vi "RUSHShoot.vi"(1 "In Cluster":T2) -> (0 "Out Cluster":T1)   [LabVIEW 2012]
panel:
  in  "Highest POT pos":dbl=4.2
  in  "Lowest POT pos":dbl=2.1
  in  "ShootPOTToPowConst":dbl=1.0
  in  "Vision Speed Const":dbl=0.75
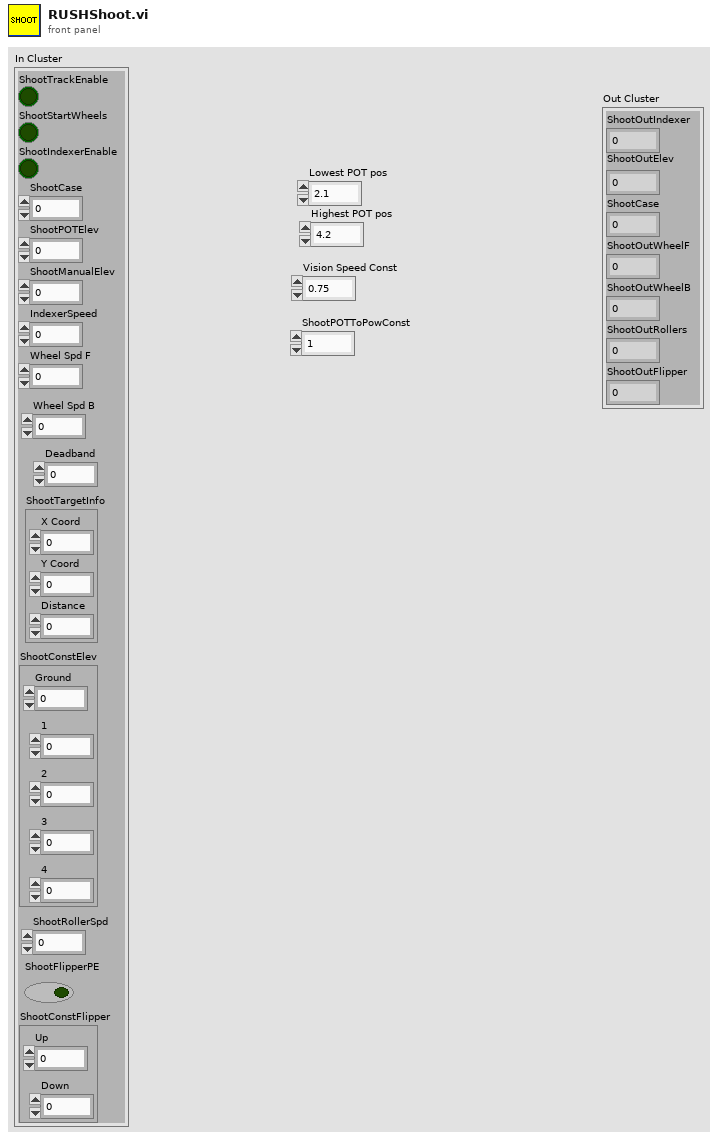
[diagram p1: front panel]
types:
  T1 = cluster{"ShootOutIndexer":dbl, "ShootOutElev":dbl, "ShootCase":dbl, "ShootOutWheelF":dbl, "ShootOutWheelB":dbl, "ShootOutRollers":dbl, "ShootOutFlipper":dbl}
  T2 = cluster{"ShootTrackEnable":bool, "ShootStartWheels":bool, "ShootIndexerEnable":bool, "ShootCase":dbl, "ShootPOTElev":dbl, "ShootManualElev":dbl, "IndexerSpeed":dbl, "Wheel Spd F":dbl, "Deadband":dbl, "ShootTargetInfo":cluster{"X Coord":dbl, "Y Coord":dbl, "Distance":dbl}, "ShootConstElev":cluster{"1":dbl, "2":dbl, "3":dbl, "4":dbl, "Ground":dbl}, "ShootRollerSpd":dbl, "ShootFlipperPE":bool, "ShootConstFlipper":cluster{"Down":dbl, "Up":dbl}, "Wheel Spd B":dbl}
  T3 = cluster{"X Coord":dbl, "Y Coord":dbl, "Distance":dbl}
  T4 = cluster{"1":dbl, "2":dbl, "3":dbl, "4":dbl, "Ground":dbl}
  T5 = cluster{"f":dbl, "y":dbl, "f":dbl, "f":dbl, "f":dbl, "f":dbl, "Down":dbl}
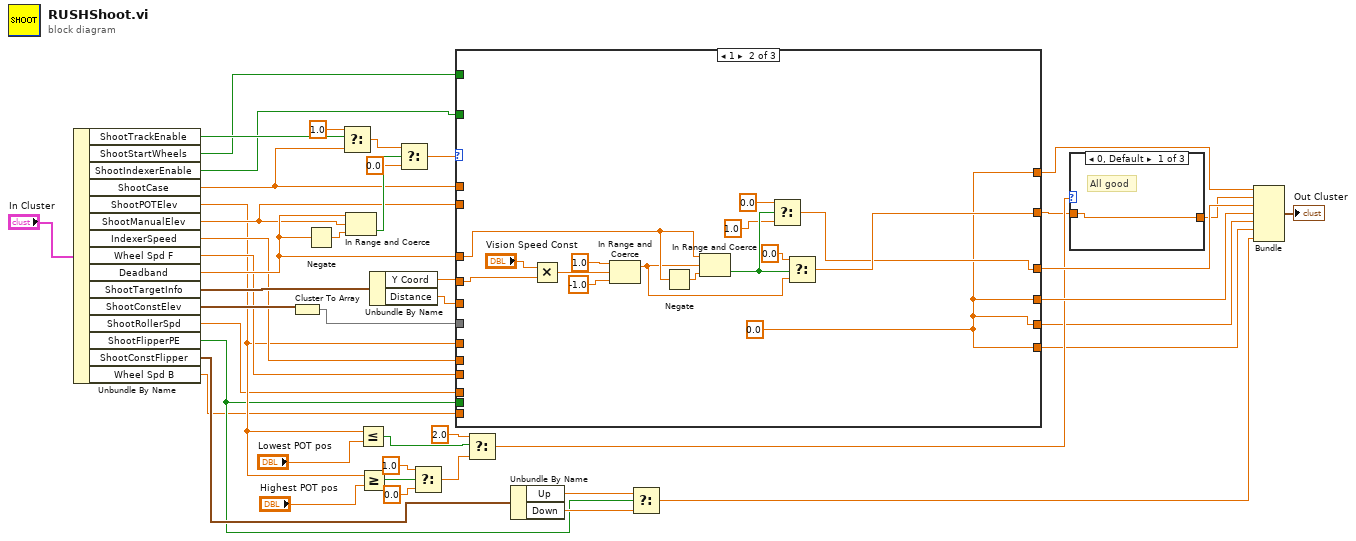
[diagram p0: block diagram]
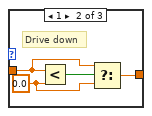
[diagram p2: hidden frame]
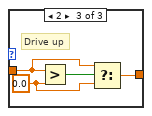
[diagram p3: hidden frame]
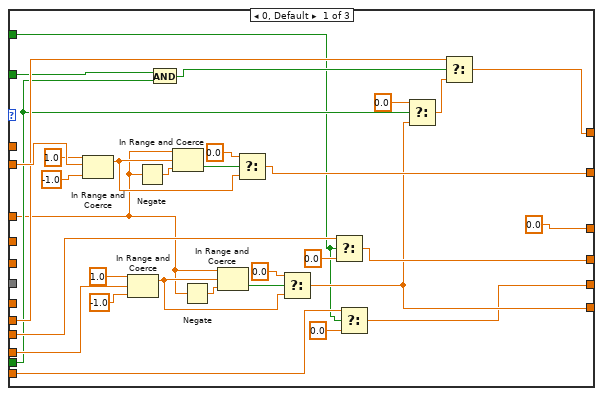
[diagram p4: hidden frame]
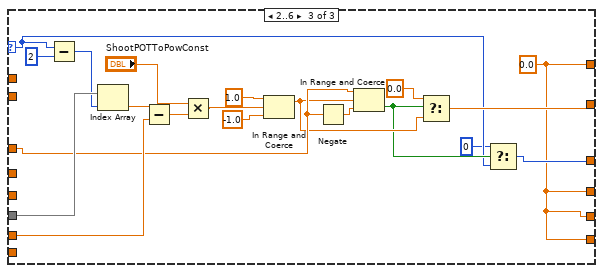
[diagram p5: hidden frame]
diagram:
  n1 = Unbundle By Name("In Cluster") -> ("ShootTrackEnable"=w44:bool, "ShootStartWheels"=w32:bool, "ShootIndexerEnable"=w31:bool, "ShootCase"=w33:dbl, "ShootPOTElev"=w21:dbl, "ShootManualElev"=w30:dbl, "IndexerSpeed"=w24:dbl, "Wheel Spd F"=w23:dbl, "Deadband"=w34:dbl, "ShootTargetInfo"=w37:T3, "ShootConstElev"=w29:T4, "ShootRollerSpd"=w10:dbl, "ShootFlipperPE"=w6:bool, "ShootConstFlipper"=w8:cluster{"Down":dbl, "Up":dbl}, "Wheel Spd B"=w5:dbl)
  n2 = Cluster To Array(cluster=w29) -> (array=w28:dbl[])
  n3 = Negate(x=w34) -> (-x=w41:dbl)
  n4 = Select(t=1.0, s=w44, f=w33) -> (s? t:f=w42:dbl)
  n5 = In Range and Coerce(upper limit=w34, x=w30, lower limit=w41) -> (In Range?=w40:bool)  [unwired: 1 out]
  n6 = Less Or Equal?(x=w21, y="Lowest POT pos") -> (x <= y?=w15:bool)
  n7 = Greater Or Equal?(x=w21, y="Highest POT pos") -> (x >= y?=w19:bool)
  n8 = Unbundle By Name(w37) -> ("Y Coord"=w36:dbl, "Distance"=w35:dbl)
  n9 = Select(t=w42, s=w40, f=0.0) -> (s? t:f=w38:dbl)
  n10 = Select(t=1.0, s=w19, f=0.0) -> (s? t:f=w16:dbl)
  n11 = case shown="1" w38 {
    selector: w38 -> [_ _ w96]
    tunnel: w36 -> [_ w91 _]
    tunnel: w35 -> [_ _ _]
    tunnel: w34 -> [w50 w86 w101]
    tunnel: [0.0 ("upper limit") w80 w94] -> w26
    tunnel: w33 -> [_ _ _]
    tunnel: [w70 w81 w98] -> w12
    tunnel: [w68 w78 w93] -> w25
    tunnel: [w77 w78 w93] -> w27
    tunnel: w32 -> [w47 _ _]
    tunnel: w31 -> [w56 _ _]
    tunnel: w30 -> [w74 _ _]
    tunnel: w28 -> [_ _ w111]
    tunnel: w21 -> [_ _ w108]
    tunnel: w24 -> [w64 _ _]
    tunnel: w23 -> [w65 _ _]
    tunnel: w10 -> [w57 _ _]
    tunnel: [w52 w78 w93] -> w3
    tunnel: w6 -> [w54 _ _]
    tunnel: w5 -> [w48 _ _]
    tunnel: [w46 w78 w93] -> w2
    frame 0, Default {
      n12 = In Range and Coerce(upper limit=1.0, x=w74, lower limit=-1.0 ("upper limit")) -> (coerced(x)=w71:dbl)  [unwired: 1 out]
      n13 = In Range and Coerce(upper limit=1.0, x=w57, lower limit=-1.0 ("upper limit")) -> (coerced(x)=w62:dbl)  [unwired: 1 out]
      n14 = Negate(x=w50) -> (-x=w75:dbl)
      n15 = And(x=w56, y=w54) -> (x .and. y?=w55:bool)
      n16 = In Range and Coerce(upper limit=w50, x=w71, lower limit=w75) -> (In Range?=w73:bool)  [unwired: 1 out]
      n17 = Negate(x=w50) -> (-x=w59:dbl)
      n18 = In Range and Coerce(upper limit=w50, x=w62, lower limit=w59) -> (In Range?=w60:bool)  [unwired: 1 out]
      n19 = Select(t=0.0, s=w73, f=w71) -> (s? t:f=w70:dbl)
      n20 = Select(t=0.0, s=w60, f=w62) -> (s? t:f=w52:dbl)
      n21 = Select(t=w65, s=w47, f=0.0 ("t")) -> (s? t:f=w68:dbl)
      n22 = Select(t=w48, s=w47, f=0.0 ("t")) -> (s? t:f=w46:dbl)
      n23 = Select(t=0.0, s=w54, f=w52) -> (s? t:f=w51:dbl)
      n24 = Select(t=w64, s=w55, f=w51) -> (s? t:f=w77:dbl)
    }
    frame 1 {
      w78 = 0.0
      n25 = Multiply(x="Vision Speed Const", y=w91) -> (x*y=w90:dbl)
      n26 = In Range and Coerce(upper limit=1.0, x=w90, lower limit=-1.0 ("upper limit")) -> (coerced(x)=w84:dbl)  [unwired: 1 out]
      n27 = Negate(x=w86) -> (-x=w87:dbl)
      n28 = In Range and Coerce(upper limit=w86, x=w84, lower limit=w87) -> (In Range?=w83:bool)  [unwired: 1 out]
      n29 = Select(t=0.0, s=w83, f=1.0) -> (s? t:f=w80:dbl)
      n30 = Select(t=0.0, s=w83, f=w84) -> (s? t:f=w81:dbl)
    }
    frame 2..6 {
      w93 = 0.0 ("f")
      n31 = Subtract(x=w96, y=2) -> (x-y=w110:i32)
      n32 = Index Array(array=w111, index=w110) -> (element=w109:dbl)
      n33 = Subtract(x=w109, y=w108) -> (x-y=w107:dbl)
      n34 = Multiply(x="ShootPOTToPowConst", y=w107) -> (x*y=w102:dbl)
      n35 = In Range and Coerce(upper limit=1.0, x=w102, lower limit=-1.0 ("upper limit")) -> (coerced(x)=w99:dbl)  [unwired: 1 out]
      n36 = Negate(x=w101) -> (-x=w103:dbl)
      n37 = In Range and Coerce(upper limit=w101, x=w99, lower limit=w103) -> (In Range?=w97:bool)  [unwired: 1 out]
      n38 = Select(t=0.0, s=w97, f=w99) -> (s? t:f=w98:dbl)
      n39 = Select(t=0, s=w97, f=w96) -> (s? t:f=w94:i32)
    }
  }
  n40 = Select(t=2.0, s=w15, f=w16) -> (s? t:f=w13:dbl)
  n41 = Unbundle By Name(w8) -> ("Up"=w7:dbl, "Down"=w9:dbl)
  n42 = Select(t=w7, s=w6, f=w9) -> (s? t:f=w4:dbl)
  n43 = case shown="0, Default" w13 {
    tunnel: w12 -> [w113 w115 w119]
    tunnel: [w113 w114 w118] -> w11
    frame 0, Default {
      # "All good"
    }
    frame 1 {
      w116 = 0.0 ("y")
      # "Drive down"
      n44 = Less?(x=w115, y=w116) -> (x < y?=w117:bool)
      n45 = Select(t=w115, s=w117, f=w116) -> (s? t:f=w114:dbl)
    }
    frame 2 {
      w120 = 0.0 ("y")
      # "Drive up"
      n46 = Greater?(x=w119, y=w120) -> (0:w121:bool)
      n47 = Select(t=w119, s=w121, f=w120) -> (s? t:f=w118:dbl)
    }
  }
  n48 = Bundle("f"=w27, "y"=w11, "f"=w26, "f"=w25, "f"=w2, "f"=w3, "Down"=w4) -> (→"Out Cluster":T5)  [unwired: 1 in]
